vi "Generate Msg Event DVR.vi"(9 "Msg":refnum<class "Msg.lvclass">, 10 "Msg Event DVR":refnum<data-value>) -> (0 "error out":errorcluster)   [LabVIEW 2021, in "jettl.lvlib"]
uses:
  jettl.lvlib
  Actor/Msg/Msg.lvclass
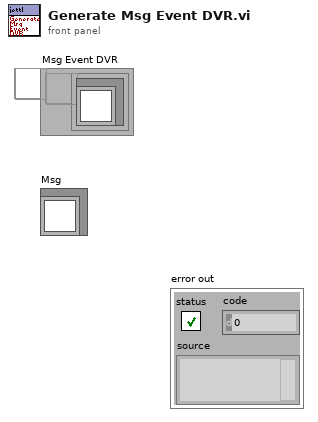
[diagram p1: front panel]
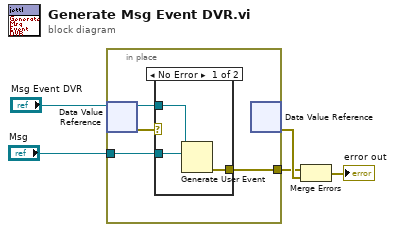
[diagram p0: block diagram]
diagram:
  n1 = in-place {
    in-place-border: "Msg" -> [w9]
    in-place-border: [w8] -> w2
    n2 = in-place-dvr #1("Msg Event DVR") -> (w7:refnum<user-event>, w6:errorcluster)
    n3 = case shown="No Error" w6 {
      selector: w6 -> [_ w13]
      tunnel: w9 -> [w11 _]
      tunnel: [w10 w13] -> w8
      tunnel: w7 -> [w12 _]
      frame No Error {
        n4 = Generate User Event(user event=w12, event data cluster=w11) -> (error out=w10:errorcluster)  [unwired: 2 in, 1 out]
      }
      frame Error {
      }
    }
    n5 = in-place-dvr #1() -> (w3:errorcluster)  [unwired: 1 in, 1 out]
  }
  n6 = Merge Errors(w2, w3) -> (→"error out":errorcluster)
